vi "calc_imaq_images_for_display.vi"(6 "Raw data in":dbl[][][](array[numeric]), 7 "Lower bounds array":dbl[](array[numeric]), 8 "error in":errorcluster, 9 "Color tables display":T2[](array[typedef])=[enum."Grayscale"], 10 "Upper bounds array":dbl[](array[numeric]), 11 "Image in":T1) -> (0 "error out":errorcluster, 3 "Image Out":T1)   [LabVIEW 2011, in "Fiberscope_library.lvlib"]
uses:
  Fiberscope_library.lvlib
  typedefs/color_palette_enum.ctl
  <vilib>/vision/Image Controls.llb/IMAQ Image.ctl
  <vilib>/vision/NI_Vision_Development_Module.lvlib
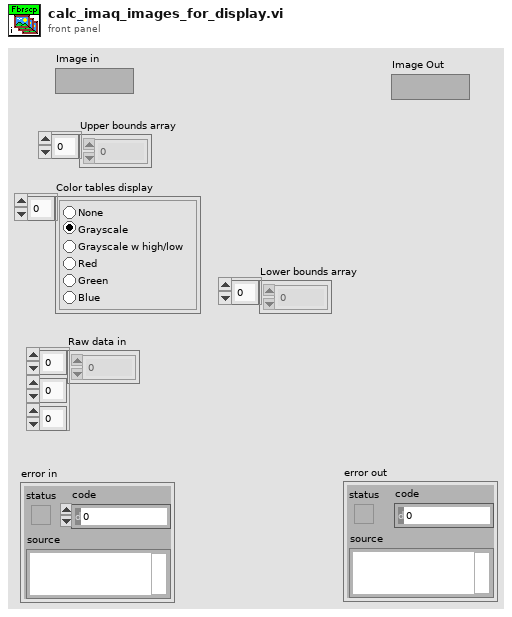
[diagram p1: front panel]
types:
  T1 = typedef "IMAQ Image.ctl" = refnum<image>
  T2 = typedef "Fiberscope_library.lvlib/color_palette_enum.ctl" = enum32{"None", "Grayscale", "Grayscale w high/low", "Red", "Green", "Blue"}
  T3 = enum32{"Average", "Min", "Max", "Clear  if < ", "Clear  if < or =", "Clear  if =", "Clear  if > or =", "Clear  if >"}
  T4 = typedef "Image Type" = u32
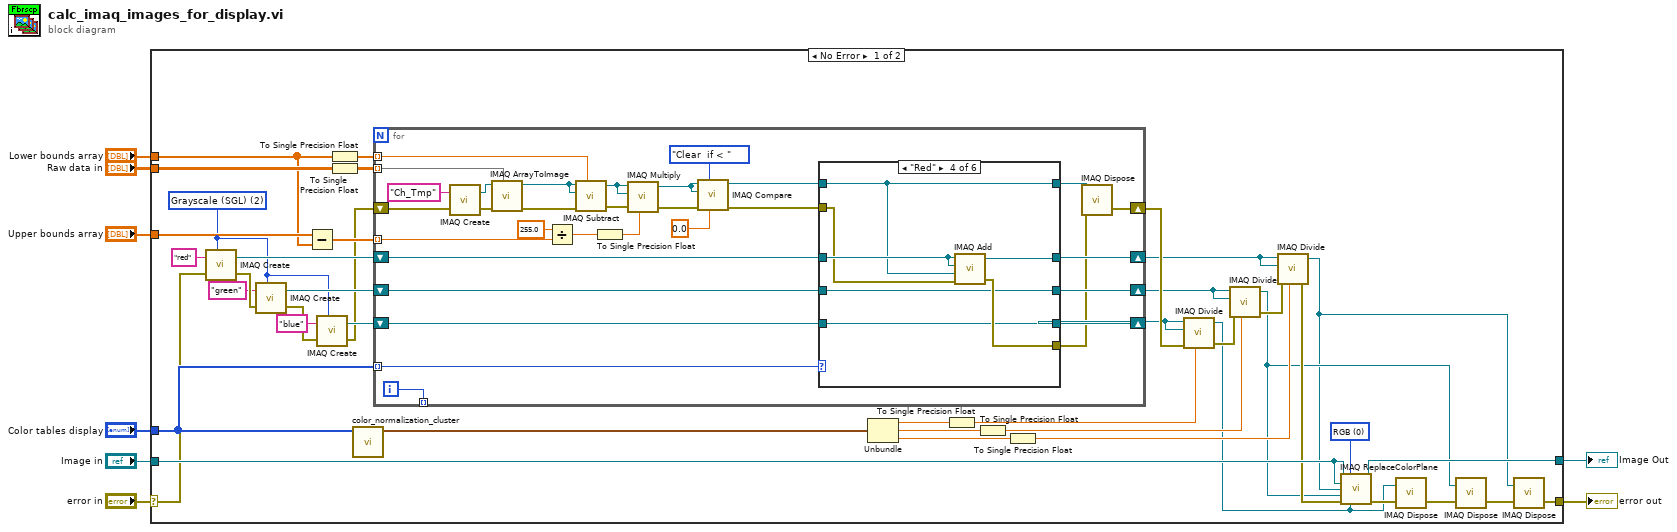
[diagram p0: block diagram]
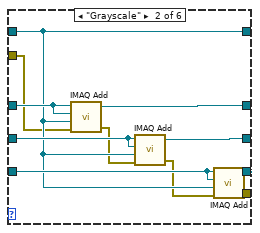
[diagram p3: hidden frame]
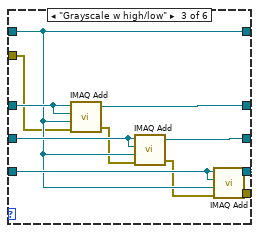
[diagram p4: hidden frame]
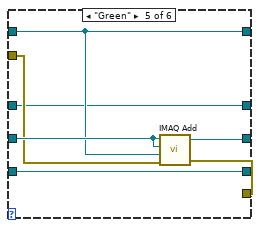
[diagram p5: hidden frame]
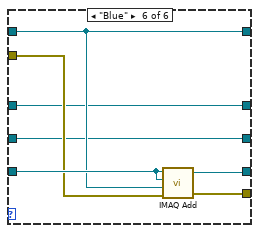
[diagram p6: hidden frame]
diagram:
  n1 = case shown="No Error" "error in" {
    selector: "error in" -> [w26 w130]
    tunnel: "Raw data in" -> [w46 _]
    tunnel: "Image in" -> [w28 w131]
    tunnel: [w30 w131] -> w6
    tunnel: [w11 w130] -> w4
    tunnel: "Upper bounds array" -> [w48 _]
    tunnel: "Color tables display" -> [w50 _]
    tunnel: "Lower bounds array" -> [w44 _]
    frame No Error {
      w16 = T4 2 items=["Grayscale (U8)", "Grayscale (I16)", "Grayscale (SGL)", "Complex (CSG)", "RGB (U32)", "HSL (U32)", "RGB (U64)", "Grayscale (U16)"] ("Image Type")
      w29 = u16 0 items=["RGB", "HSL", "HSV", "HSI"] ("Color Mode")
      n2 = call "IMAQ Create"("Image Name"="red", "Image Type"=w16, "error in (no error)"=w26) -> ("New Image"=w24:T1, "error out"=w22:errorcluster)  [unwired: 2 in]
      n3 = call "IMAQ Create"("Image Name"="green", "Image Type"=w16, "error in (no error)"=w22) -> ("New Image"=w23:T1, "error out"=w19:errorcluster)  [unwired: 2 in]
      n4 = Subtract(x=w48, y=w44) -> (x-y=w47:dbl[])
      n5 = call "IMAQ Create"("Image Name"="blue", "Image Type"=w16, "error in (no error)"=w19) -> ("New Image"=w20:T1, "error out"=w17:errorcluster)  [unwired: 2 in]
      n6 = To Single Precision Float(number=w44) -> (single precision float=w43:sgl[])
      n7 = To Single Precision Float(number=w46) -> (single precision float=w45:sgl[][][])
      n8 = call "color_normalization_cluster.vi"("Color tables array"=w50) -> ("Normalization cluster"=w49:cluster{"[0]":dbl, "[1]":dbl, "[2]":dbl})  [unwired: 10 in]
      n9 = for {
        tunnel: w45 -> [w79] mode=indexing
        tunnel: w50 -> [w67] mode=indexing
        shift-right: [w61] -> w33
        shift-left: w24 -> [w66]
        shift-right: [w60] -> w36
        shift-left: w23 -> [w65]
        shift-right: [w59] -> w41
        shift-left: w20 -> [w64]
        tunnel: w43 -> [w76] mode=indexing
        tunnel: w47 -> [w80] mode=indexing
        shift-right: [w52] -> w42
        shift-left: w17 -> [w56]
        tunnel: [w51] -> _ mode=indexing
        i -> [w51]
        n10 = call "IMAQ Create"("Image Name"="Ch_Tmp", "error in (no error)"=w56) -> ("New Image"=w58:T1, "error out"=w57:errorcluster)  [unwired: 3 in]
        n11 = call "IMAQ ArrayToImage"("Image Pixels (Float)"=w79, "error in (no error)"=w57, "Image"=w58) -> ("error out"=w77:errorcluster, "Image Out"=w78:T1)  [unwired: 7 in]
        n12 = Divide(x=255.0, y=w80) -> (x/y=w73:dbl)
        n13 = call "IMAQ Subtract"("Image Src A"=w78, "Constant"=w76, "Image Dst"=w78, "error in (no error)"=w77) -> ("Image Dst Out"=w74:T1, "error out"=w75:errorcluster)  [unwired: 3 in]
        n14 = To Single Precision Float(number=w73) -> (single precision float=w72:sgl)
        n15 = call "IMAQ Multiply"("Image Src A"=w74, "Constant"=w72, "Image Dst"=w74, "error in (no error)"=w75) -> ("Image Dst Out"=w70:T1, "error out"=w71:errorcluster)  [unwired: 3 in]
        n16 = call "IMAQ Compare"("Constant"=sgl 0.0, "Operator"=T3."Clear  if < ", "error in (no error)"=w71, "Image Dst"=w70, "Image Src A"=w70) -> ("error out"=w62:errorcluster, "Image Dst Out"=w63:T1)  [unwired: 5 in]
        n17 = case shown="\"Red\"" w67 {
          tunnel: w66 -> [w86 w97 w108 w115 w118 w123]
          tunnel: w65 -> [w85 w96 w107 w110 w122 w124]
          tunnel: w64 -> [w84 w95 w106 w109 w117 w129]
          tunnel: w63 -> [w82 w94 w105 w114 w121 w128]
          tunnel: w62 -> [w83 w90 w101 w113 w120 w127]
          tunnel: [w86 w93 w104 w111 w118 w123] -> w61
          tunnel: [w85 w92 w103 w110 w119 w124] -> w60
          tunnel: [w84 w91 w102 w109 w117 w126] -> w59
          tunnel: [w83 w87 w98 w112 w116 w125] -> w53
          tunnel: [w82 w94 w105 w114 w121 w128] -> w54
          frame "None", Default {
          }
          frame "Grayscale" {
            n18 = call "IMAQ Add"("Image Src A"=w97, "Image Dst"=w97, "Image Src B"=w94, "error in (no error)"=w90) -> ("Image Dst Out"=w93:T1, "error out"=w89:errorcluster)  [unwired: 3 in]
            n19 = call "IMAQ Add"("Image Src A"=w96, "Image Dst"=w96, "Image Src B"=w94, "error in (no error)"=w89) -> ("Image Dst Out"=w92:T1, "error out"=w88:errorcluster)  [unwired: 3 in]
            n20 = call "IMAQ Add"("Image Src A"=w95, "Image Dst"=w95, "Image Src B"=w94, "error in (no error)"=w88) -> ("Image Dst Out"=w91:T1, "error out"=w87:errorcluster)  [unwired: 3 in]
          }
          frame "Grayscale w high/low" {
            n21 = call "IMAQ Add"("Image Src A"=w108, "Image Dst"=w108, "Image Src B"=w105, "error in (no error)"=w101) -> ("Image Dst Out"=w104:T1, "error out"=w100:errorcluster)  [unwired: 3 in]
            n22 = call "IMAQ Add"("Image Src A"=w107, "Image Dst"=w107, "Image Src B"=w105, "error in (no error)"=w100) -> ("Image Dst Out"=w103:T1, "error out"=w99:errorcluster)  [unwired: 3 in]
            n23 = call "IMAQ Add"("Image Src A"=w106, "Image Dst"=w106, "Image Src B"=w105, "error in (no error)"=w99) -> ("Image Dst Out"=w102:T1, "error out"=w98:errorcluster)  [unwired: 3 in]
          }
          frame "Red" {
            n24 = call "IMAQ Add"("Image Src A"=w115, "Image Dst"=w115, "Image Src B"=w114, "error in (no error)"=w113) -> ("Image Dst Out"=w111:T1, "error out"=w112:errorcluster)  [unwired: 3 in]
          }
          frame "Green" {
            n25 = call "IMAQ Add"("Image Src A"=w122, "Image Dst"=w122, "Image Src B"=w121, "error in (no error)"=w120) -> ("Image Dst Out"=w119:T1, "error out"=w116:errorcluster)  [unwired: 3 in]
          }
          frame "Blue" {
            n26 = call "IMAQ Add"("Image Src A"=w129, "Image Dst"=w129, "Image Src B"=w128, "error in (no error)"=w127) -> ("Image Dst Out"=w126:T1, "error out"=w125:errorcluster)  [unwired: 3 in]
          }
        }
        n27 = call "IMAQ Dispose"("Image"=w54, "error in (no error)"=w53) -> ("error out"=w52:errorcluster)  [unwired: 4 in]
      }
      n28 = Unbundle(w49) -> ("[0]"=w40:dbl, "[1]"=w38:dbl, "[2]"=w37:dbl)
      n29 = To Single Precision Float(number=w40) -> (single precision float=w39:sgl)
      n30 = To Single Precision Float(number=w38) -> (single precision float=w34:sgl)
      n31 = To Single Precision Float(number=w37) -> (single precision float=w31:sgl)
      n32 = call "IMAQ Divide"("Image Src A"=w41, "Constant"=w39, "Image Dst"=w41, "error in (no error)"=w42) -> ("Image Dst Out"=w14:T1, "error out"=w35:errorcluster)  [unwired: 3 in]
      n33 = call "IMAQ Divide"("Image Src A"=w36, "Constant"=w34, "Image Dst"=w36, "error in (no error)"=w35) -> ("Image Dst Out"=w10:T1, "error out"=w32:errorcluster)  [unwired: 3 in]
      n34 = call "IMAQ Divide"("Image Src A"=w33, "Constant"=w31, "Image Dst"=w33, "error in (no error)"=w32) -> ("Image Dst Out"=w9:T1, "error out"=w27:errorcluster)  [unwired: 3 in]
      n35 = call "IMAQ ReplaceColorPlane"("Image Src"=w28, "Color Mode"=w29, "Image Dst"=w28, "Red or Hue Plane"=w9, "Green or Sat Plane"=w10, "error in (no error)"=w27, "Blue or Luma or Val or Inten Plane"=w14) -> ("Image Dst Out"=w30:T1, "error out"=w15:errorcluster)  [unwired: 7 in]
      n36 = call "IMAQ Dispose"("Image"=w14, "error in (no error)"=w15) -> ("error out"=w13:errorcluster)  [unwired: 4 in]
      n37 = call "IMAQ Dispose"("Image"=w10, "error in (no error)"=w13) -> ("error out"=w12:errorcluster)  [unwired: 4 in]
      n38 = call "IMAQ Dispose"("Image"=w9, "error in (no error)"=w12) -> ("error out"=w11:errorcluster)  [unwired: 4 in]
    }
    frame Error {
    }
  }
  "Image Out" <- w6
  "error out" <- w4
